vi "setTemperature.vi"(8 "error in (no error)":errorcluster, 10 "setPoint":dbl, 11 "ProEM_WinX32 in":refnum<class "ProEM_WinX32.lvclass">) -> (0 "error out":errorcluster, 3 "ProEM_WinX32 out":refnum<class "ProEM_WinX32.lvclass">)   [LabVIEW 2011, in "Hardware.lvlib" / "Channels.lvlib" / "ProEM_WinX32.lvclass"]
uses:
  ProEM_WinX32.lvclass
  Camera/Camera.lvclass
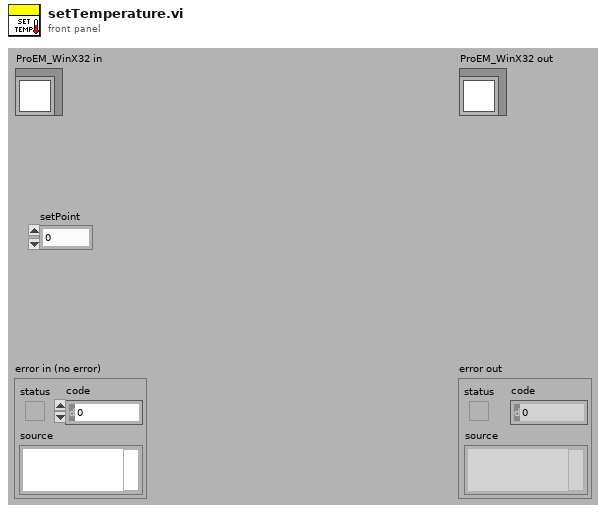
[diagram p1: front panel]
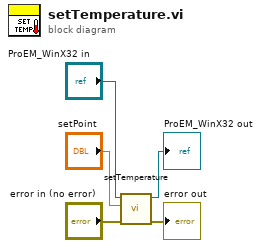
[diagram p0: block diagram]
diagram:
  n1 = call-parent "setTemperature.vi"("error in (no error)"="error in (no error)", "setPoint"="setPoint", "Camera in"="ProEM_WinX32 in") -> ("error out"=→"error out":errorcluster, "Camera out"=→"ProEM_WinX32 out":refnum<class "ProEM_WinX32.lvclass">)  [unwired: 7 in]
